vi "ReadZero.vi"(2 "error in":errorcluster, 3 "zero In":dbl) -> (0 "error out":errorcluster, 1 "zero Out":dbl)   [LabVIEW 2013]
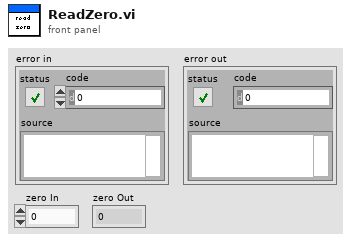
[diagram p1: front panel]
types:
  T1 = enum16{"open", "replace", "create", "open or create", "replace or create", "replace or create with confirmation"}
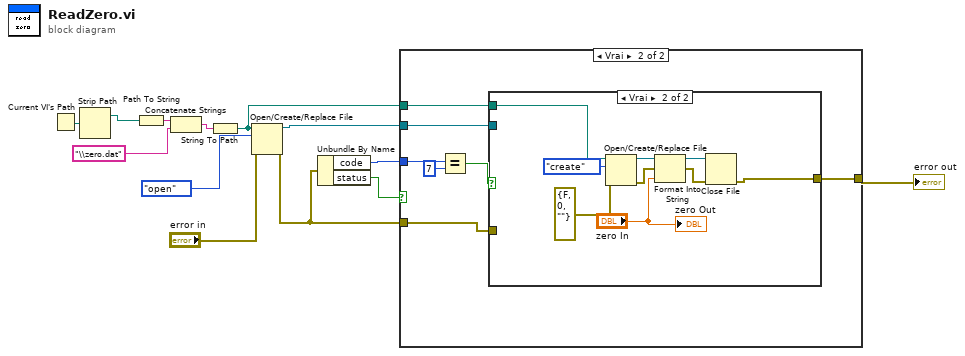
[diagram p0: block diagram]
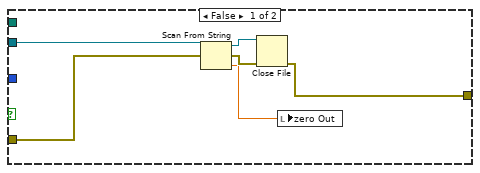
[diagram p2: hidden frame]
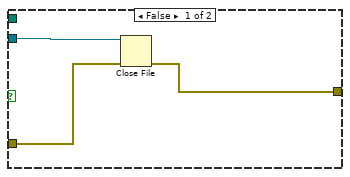
[diagram p3: hidden frame]
diagram:
  n1 = Current VI's Path() -> (path=w13:path)
  n2 = Strip Path(path=w13) -> (stripped path=w12:path)  [unwired: 1 out]
  n3 = Path To String(path=w12) -> (string=w11:string)
  n4 = Concatenate Strings(w11, "\\zero.dat" ("chaîne")) -> (w10:string)
  n5 = String To Path(string=w10) -> (path=w1:path)
  n6 = Open/Create/Replace File(file path (use dialog)=w1, error in="error in", operation (0:open)=T1."open") -> (refnum out=w8:refnum<file>, error out=w4:errorcluster)  [unwired: 3 in, 1 out]
  n7 = Unbundle By Name(w4) -> ("code"=w2:i32, "status"=w3:bool)
  n8 = case shown="Vrai" w3 {
    tunnel: w8 -> [w19 w26]
    tunnel: w4 -> [w18 w25]
    tunnel: [w15 w24] -> w5
    tunnel: w2 -> [_ w23]
    tunnel: w1 -> [_ w20]
    frame False {
      n9 = Scan From String(w19, w18) -> (w17:refnum<file>, w16:errorcluster, output 1=w14:dbl)  [unwired: 2 in]
      n10 = Close File(refnum=w17, error in=w16) -> (error out=w15:errorcluster)  [unwired: 1 out]
      n11 = local write "zero Out"(w14) -> ()
    }
    frame True {
      n12 = Equal?(x=w23, y=7) -> (x = y?=w21:bool)
      n13 = case shown="Vrai" w21 {
        tunnel: w26 -> [w29 _]
        tunnel: w25 -> [w28 _]
        tunnel: [w27 w32] -> w24
        tunnel: w20 -> [_ w38]
        frame False {
          n14 = Close File(refnum=w29, error in=w28) -> (error out=w27:errorcluster)  [unwired: 1 out]
        }
        frame True {
          n15 = Open/Create/Replace File(file path (use dialog)=w38, error in=errorcluster {"status"=FALSE, "code"=0, "source"=""} ("entrée d'erreur"), operation (0:open)=T1."create") -> (refnum out=w35:refnum<file>, error out=w36:errorcluster)  [unwired: 3 in, 1 out]
          n16 = Format Into String(initial string=w35, error in=w36, "zero In") -> (resulting string=w33:refnum<file>, error out=w34:errorcluster)  [unwired: 1 in]
          n17 = Close File(refnum=w33, error in=w34) -> (error out=w32:errorcluster)  [unwired: 1 out]
          "zero Out" <- "zero In"
        }
      }
    }
  }
  "error out" <- w5
